vi "Test Array to Map.vi"() -> ()   [LabVIEW 2020]
uses:
  7ad088f9-4a2d-4d77-8d6b-6665f0c03ec1.vi
  7ad088f9-4a2d-4d77-8d6b-6665f0c03ec1.vi/b0178052-0c48-4c9a-874f-40b592e34ac5.vi
  <vilib>/addons/_JKI Toolkits/Caraya/classes/Assert/Assert.lvclass
panel:
  out "error out":errorcluster
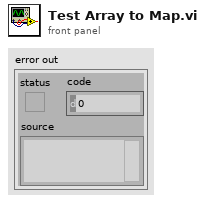
[diagram p1: front panel]
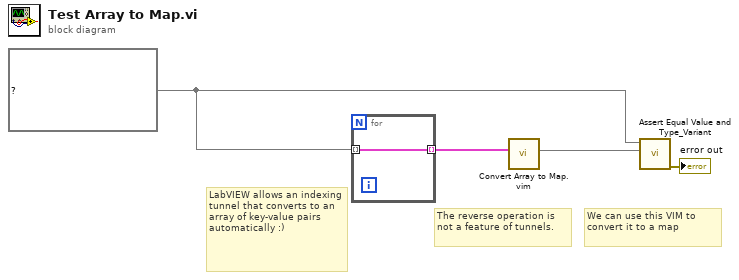
[diagram p0: block diagram]
diagram:
  w2 = map{i32, cluster{"bool":bool, "string":string}} {0={"bool"=FALSE, "string"="zero"}, 1={"bool"=TRUE, "string"="one"}} ("map out")
  # "We can use this VIM to convert it to a map"
  # "The reverse operation is not a feature of tunnels."
  # "LabVIEW allows an indexing tunnel that converts to an array of key-value pairs automatically :)"
  n1 = for {
    tunnel: [w5] -> w4 mode=indexing
    tunnel: w2 -> [w5] mode=indexing
  }
  n2 = call "Convert Array to Map.vim"("array"=w4) -> ("map"=w3:map{i32, cluster{"bool":bool, "string":string}})  [unwired: 10 in]
  n3 = call <vilib>:"Assert Equal Value and Type_Variant.vi"("Y"=w3, "X"=w2) -> ("error out"=→"error out":errorcluster)  [unwired: 9 in]
